vi "xPacket_v1.vi"(1 "addrs values":i32, 2 "addrs":i32, 3 "no. addrs":i32, 4 "command":string) -> (0 "String":string)   [LabVIEW 2018]
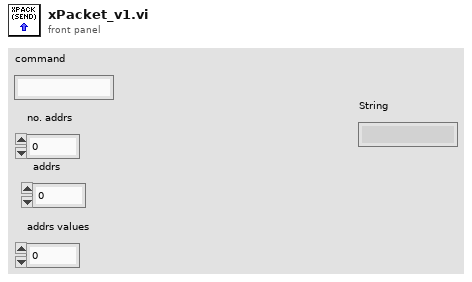
[diagram p1: front panel]
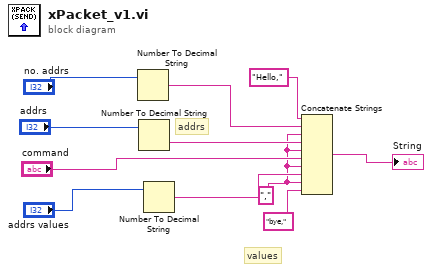
[diagram p0: block diagram]
diagram:
  w1 = "," ("string")
  # "values"
  # "addrs"
  n1 = Number To Decimal String(number="no. addrs") -> (decimal integer string=w4:string)  [unwired: 1 in]
  n2 = Number To Decimal String(number="addrs") -> (decimal integer string=w3:string)  [unwired: 1 in]
  n3 = Number To Decimal String(number="addrs values") -> (decimal integer string=w11:string)  [unwired: 1 in]
  n4 = Concatenate Strings("Hello," ("string"), w4, w1, w3, w1, "command", w1, w11, w1, "bye," ("string")) -> (→"String":string)
